vi "Read Browse Button_Disabled.vi"(9 "Path in":refnum<class "Path.lvclass">) -> (3 "Path out":refnum<class "Path.lvclass">, 4 "Browse Button:Disabled":u8)   [LabVIEW 2014, in "Path.lvclass"]
uses:
  Path.lvclass
  Path.lvclass/Path.ctl
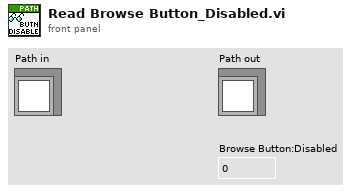
[diagram p1: front panel]
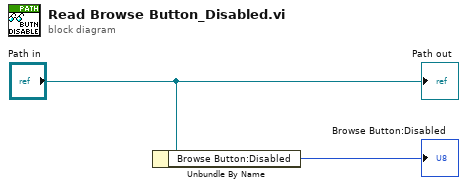
[diagram p0: block diagram]
diagram:
  n1 = Unbundle By Name("Path in") -> ("Browse Button:Disabled"=→"Browse Button:Disabled":u8)
  "Path out" <- "Path in"
